vi "Combo Recurse.vi"(4 "Level":i32, 6 "All Values":variant[](array[variant]), 7 "Map In":map{string, variant}(c390), 9 "All Inputs":string[](array[string]), 10 "To Add":variant[](array[variant]), 11 "key":string) -> (3 "Maps Out":map{string, variant}[](array[numeric]))   [LabVIEW 2020, in "Approval Tests.lvlib"]
uses:
  Approval Tests.lvlib
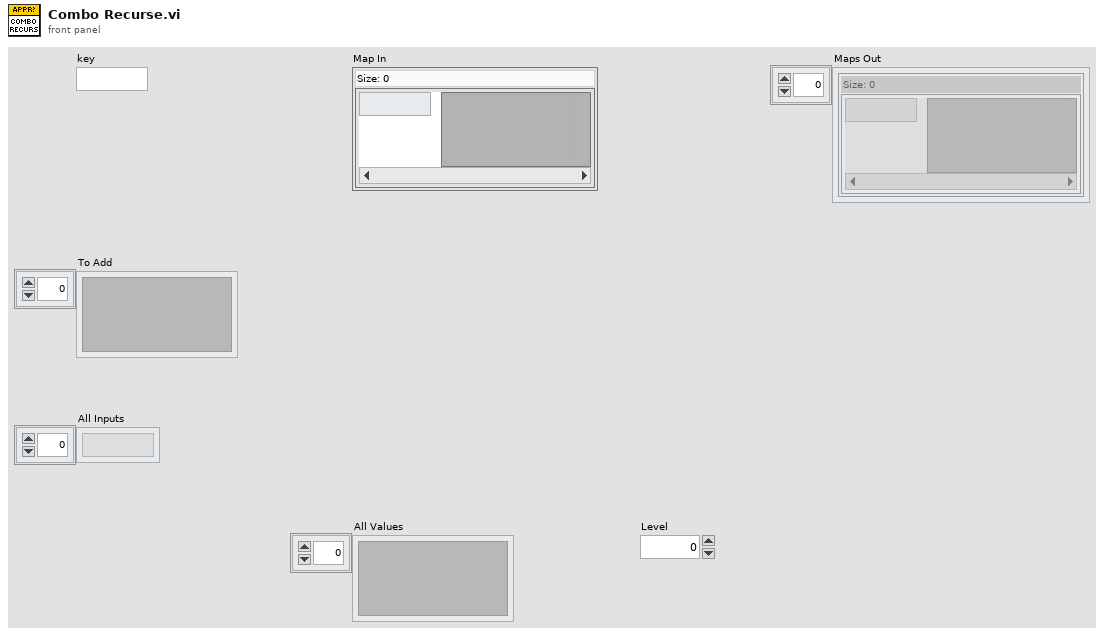
[diagram p1: front panel]
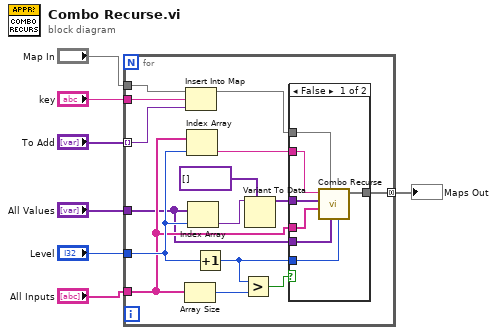
[diagram p0: block diagram]
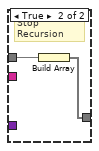
[diagram p2: hidden frame]
diagram:
  n1 = for {
    tunnel: "To Add" -> [w20] mode=indexing
    tunnel: "Map In" -> [w22]
    tunnel: [w14] -> w2 mode=concatenating
    tunnel: "key" -> [w21]
    tunnel: "All Values" -> [w9]
    tunnel: "All Inputs" -> [w10]
    tunnel: "Level" -> [w17]
    n2 = Array Size(array=w10) -> (size(s)=w16:i32)
    n3 = Insert Into Map(map in=w22, key=w21, value=w20) -> (map out=w13:map{string, variant})  [unwired: 2 out]
    n4 = Index Array(array=w10, index=w17) -> (element=w12:string)
    n5 = Index Array(array=w9, index=w17) -> (element=w19:variant)
    n6 = Increment(x=w17) -> (x+1=w8:i32)
    n7 = Greater?(x=w8, y=w16) -> (0:w15:bool)
    n8 = Variant To Data(type=variant[] [], Variant=w19) -> (data=w11:variant[])  [unwired: 1 in, 1 out]
    n9 = case shown="False" w15 {
      tunnel: [w29 w30] -> w14
      tunnel: w13 -> [w28 w31]
      tunnel: w12 -> [w27 _]
      tunnel: w11 -> [w26 _]
      tunnel: w10 -> [w25 _]
      tunnel: w9 -> [w24 _]
      tunnel: w8 -> [w23 _]
      frame False {
        n10 = call "Combo Recurse.vi"("Level"=w23, "All Values"=w24, "Map In"=w28, "All Inputs"=w25, "To Add"=w26, "key"=w27) -> ("Maps Out"=w29:map{string, variant}[])  [unwired: 5 in]
      }
      frame True {
        # "Stop Recursion"
        n11 = Build Array(w31) -> (w30:map{string, variant}[])
      }
    }
  }
  "Maps Out" <- w2
